vi "fault daignosis.vi"() -> ()   [LabVIEW 2023]
uses:
  <vilib>/Ngene/Deep Learning Toolkit/Toolkit/NN_Train/Controls/NN_Train_Params.ctl
  <vilib>/Ngene/Deep Learning Toolkit/Toolkit/NN_Train/Controls/NN_Train_Optimizer.ctl
  <vilib>/Ngene/Deep Learning Toolkit/Toolkit/NN_Train/Controls/NN_Train_Data_Sampling.ctl
  <vilib>/Ngene/Deep Learning Toolkit/Toolkit/NN_Train/Controls/NN_LR_Policy_Cfg.ctl
  <vilib>/Ngene/Deep Learning Toolkit/Toolkit/NN_Train/Controls/NN_LR_Policy_Type.ctl
  <vilib>/Ngene/Deep Learning Toolkit/Toolkit/NN_Train/Controls/NN_Train_Session_Data.ctl
  <vilib>/Ngene/Deep Learning Toolkit/Toolkit/NN_Network/Controls/NN_Device.ctl
  <vilib>/Ngene/Deep Learning Toolkit/Toolkit/NN_Data/API/DataSet/DataSet_Types/NN_DataSets_All(In3D_Out1D).ctl
  <vilib>/Ngene/Deep Learning Toolkit/Toolkit/NN_Data/API/DataSet/DataSet_Types/NN_DataSet(In3D_Out1D).ctl
  <vilib>/Ngene/Deep Learning Toolkit/Toolkit/NN_Data/Controls/DataRef_Types/2D/NN_Data_ref(2D_SGL).ctl
  <vilib>/Ngene/Deep Learning Toolkit/Toolkit/NN_Data/API/NN_Dims(C,H,W).ctl
  <vilib>/Ngene/Deep Learning Toolkit/Toolkit/NN_Layers/Layers/FC/Controls/NN_Layer_Config(FC).ctl
  <vilib>/Ngene/Deep Learning Toolkit/Toolkit/NN_Layers/Layers/BatchNorm/Controls/NN_BN_Params.ctl
  <vilib>/Ngene/Deep Learning Toolkit/Toolkit/NN_Activations/Controls/NN_Activation_Type.ctl
  <vilib>/Ngene/Deep Learning Toolkit/Toolkit/NN_Layers/Controls/NN_Layer_Init_Params.ctl
  <vilib>/Ngene/Deep Learning Toolkit/Toolkit/NN_Layers/Controls/NN_Layer_Weight_Init_Type.ctl
  <vilib>/Ngene/Deep Learning Toolkit/Toolkit/NN_Layers/Layers/Conv2D/Controls/NN_Layer_Config(Conv2D).ctl
  <vilib>/Ngene/Deep Learning Toolkit/Toolkit/NN_Layers/Layers/Conv2D/Controls/NN_Layer_Params(Conv2D).ctl
  <vilib>/Ngene/Deep Learning Toolkit/Toolkit/NN_Layers/Layers/Conv2D/Controls/NN_Conv2D_Padding_Type.ctl
  <vilib>/Ngene/Deep Learning Toolkit/Toolkit/NN_Layers/Layers/Pool/Controls/NN_Layer_Config(Pool).ctl
  <vilib>/Ngene/Deep Learning Toolkit/Toolkit/NN_Data/API/NN_Dims(V,H).ctl
  <vilib>/Ngene/Deep Learning Toolkit/Toolkit/NN_Layers/Layers/Activation/Controls/NN_Layer_Config(Activation).ctl
  <vilib>/Ngene/Deep Learning Toolkit/Toolkit/NN_Network/Controls/NN_Save_Before_Destroy_Options.ctl
  <vilib>/Ngene/Deep Learning Toolkit/Toolkit/NN_Layers/Layers/Input/Controls/NN_Layer_Config(Input3D).ctl
  <vilib>/Ngene/Deep Learning Toolkit/Toolkit/NN_Data/Controls/NN_Data_type.ctl
  <vilib>/Ngene/Deep Learning Toolkit/Toolkit/NN_Layers/Layers/Input/NN_Layer_Create(Input3D).vi
  <vilib>/Ngene/Deep Learning Toolkit/Toolkit/NN_Layers/Layers/Conv2D/NN_Layer_Create(Conv2D).vi
  <vilib>/Ngene/Deep Learning Toolkit/Toolkit/NN_Layers/Layers/Activation/NN_Layer_Create(Activation).vi
  <vilib>/Ngene/Deep Learning Toolkit/Toolkit/NN_Layers/Layers/Pool/NN_Layer_Create(maxPool).vi
  <vilib>/Ngene/Deep Learning Toolkit/Toolkit/NN_Layers/Layers/Flatten/NN_Layer_Create(Flatten).vi
  <vilib>/Ngene/Deep Learning Toolkit/Toolkit/NN_Layers/Layers/FC/NN_Layer_Create(FC).vi
  <vilib>/Ngene/Deep Learning Toolkit/Toolkit/NN_Layers/Layers/SoftMax/NN_Layer_Create(SoftMax).vi
  <vilib>/Ngene/Deep Learning Toolkit/Toolkit/NN_Train/Loss_Functions/NN_Set_Loss(CrossEntropy).vi
  <vilib>/Ngene/Deep Learning Toolkit/Toolkit/NN_Network/subVIs/NN_Predict/NN_Predict(In3D_Out1D).vi
  <vilib>/Ngene/Deep Learning Toolkit/Toolkit/NN_Train/Eval_Loss/NN_Eval_Test_Error_Loss/NN_Eval(In3D_Out1D).vi
  <vilib>/Ngene/Deep Learning Toolkit/Toolkit/NN_Train/Eval_Loss/NN_Calc_Cofusion_Matrix/NN_Calc_Confusion_Matrix(In3D_Out1D).vi
  <vilib>/Ngene/Deep Learning Toolkit/Toolkit/NN_Data/subVIs/Dataset_Destroy/NN_Dataset_Destroy(In3D_Out1D).vi
  <vilib>/Ngene/Deep Learning Toolkit/Toolkit/Deep_Learning_Toolkit_by_Ngene.lvlib
  <vilib>/ptbypt/NI_PtbyPt.lvlib
panel:
  out "Dataset":T1={"Train"={"Inputs Ref."=variant(refnum<data-value> refnum), "Outputs Ref."=refnum, "Dataset_Size"=0, "Dims_In"={"C"=0, "H"=0, "W"=0}, "Dims_Out"=0, "Labels"=[], "File Paths"=[], "Custom_Data"=variant}, "Validation"={"Inputs Ref."=variant(refnum<data-value> refnum), "Outputs Ref."=refnum, "Dataset_Size"=0, "Dims_In"={"C"=0, "H"=0, "W"=0}, "Dims_Out"=0, "Labels"=[], "File Paths"=[], "Custom_Data"=variant}, "Test"={"Inputs Ref."=variant(refnum<data-value> refnum), "Outputs Ref."=refnum, "Dataset_Size"=0, "Dims_In"={"C"=0, "H"=0, "W"=0}, "Dims_Out"=0, "Labels"=[], "File Paths"=[], "Custom_Data"=variant}}
  in  "Tab Control":enum32{"Model train", "Prediction"}(tab)
  in  "Start Training":bool
  in  "Train dataset path":path=path "E:/其他工作/Labviewpy联合开发/CWRU_Result/bmp_dataset_32x32/train"
  in  "NN_Train_Params":T5={"Optimizer"=enum."Adam", "Beta_1"=0.9, "Beta_2"=0.999, "Weight Decay(L1)"=0.0, "Weight Decay(L2)"=0.0001, "Data_Sampling"=enum."Random"}
  in  "Eval":bool
  out "Confusion Matrix":string[][](table)=[["1500", "0", "0", "0", "0", "0", "1.0000"], ["0", "1492", "0", "0", "8", "0", "0.9947"], ["0", "0", "1498", "0", "0", "2", "0.9987"], ["0", "0", "0", "1423", "68", "9", "0.9487"], ["0", "0", "0", "78", "1411", "11", "0.9407"], ["0", "0", "40", "3", "2", "1455", "0.9700"], ["1.0000", "1.0000", "0.9740", "0.9461", "0.9476", "0.9851", ""]]
  out "Test Loss":sgl=0.121348076 format="%#.6g"
  out "Test Error":sgl=0.024555556 format="%#.6g"
  in  "LR Update Policy":T8={"Policy_Type"=enum."Step", "LR0"=0.001, "k"=200.0, "WarmUp_Policy"=enum."Ramp", "WarmUp_Iter"=0, "WarmUp_Ratio"=1.0} {"WarmUp_Ratio" min=1; "WarmUp_Iter" min=1; "LR0" format="%.7f"}
  out "Loss Graphs":cluster{"Loss":sgl, "mean":dbl, "mean":dbl}(graph)={"Loss"=0.33578137, "mean"=0.2513088881969452, "mean"=0.3710270822048187}
  in  "Stop Training":bool
  in  "Test dataset path":path=path "E:/其他工作/Labviewpy联合开发/CWRU_Result/bmp_dataset_32x32/test"
  out "Session Data":T10={"Epochs"=251.7248, "Tot_Iter"=58998, "LR"=5e-06, "LR_iter"=58999}
  out "Time_Elapsed":dbl=138.95477960000062 format="%<%H:%M:%S>t"
  out "Training Loss":sgl=0.21247883 format="%#.6g"
  in  "NN_Device 2":T11=enum."GPU"
  in  "Datain":bool
  out "Loss":dbl=0.46153685450553894
  out "Error Rate":dbl=0.15330000221729279
  in  "NN_Device":T11=enum."GPU"
  in  "Weight File Path":path=path "E:/其他工作/Labviewpy联合开发/working/Fault_Classifier/Fault_Classifier_weights_26_05_08__18_01_11.bin"
  in  "Network Configuration File Path":path=path "E:/其他工作/Labviewpy联合开发/working/Fault_Classifier/Fault_Classifier_net_cfg_26_05_08__18_01_11.cfg"
  out "Confusion Matrix 3":string[][](table)=[["850", "4", "40", "7", "12", "1", "0", "13", "42", "31", "0.8500"], ["14", "919", "1", "1", "0", "0", "2", "2", "8", "53", "0.9190"], ["38", "1", "779", "24", "58", "29", "51", "11", "7", "2", "0.7790"], ["13", "3", "56", "658", "47", "132", "56", "20", "10", "5", "0.6580"], ["4", "3", "39", "19", "866", "10", "23", "34", "2", "0", "0.8660"], ["7", "2", "32", "101", "32", "778", "16", "26", "2", "4", "0.7780"], ["6", "3", "30", "23", "17", "12", "902", "2", "4", "1", "0.9020"], ["8", "0", "16", "24", "50", "24", "2", "870", "2", "4", "0.8700"], ["43", "13", "7", "4", "4", "3", "4", "1", "909", "12", "0.9090"], ["10", "26", "4", "8", "1", "1", "2", "4", "8", "936", "0.9360"], ["0.8560", "0.9435", "0.7759", "0.7572", "0.7967", "0.7859", "0.8526", "0.8850", "0.9145", "0.8931", ""]]
  in  "Start Prediction":bool
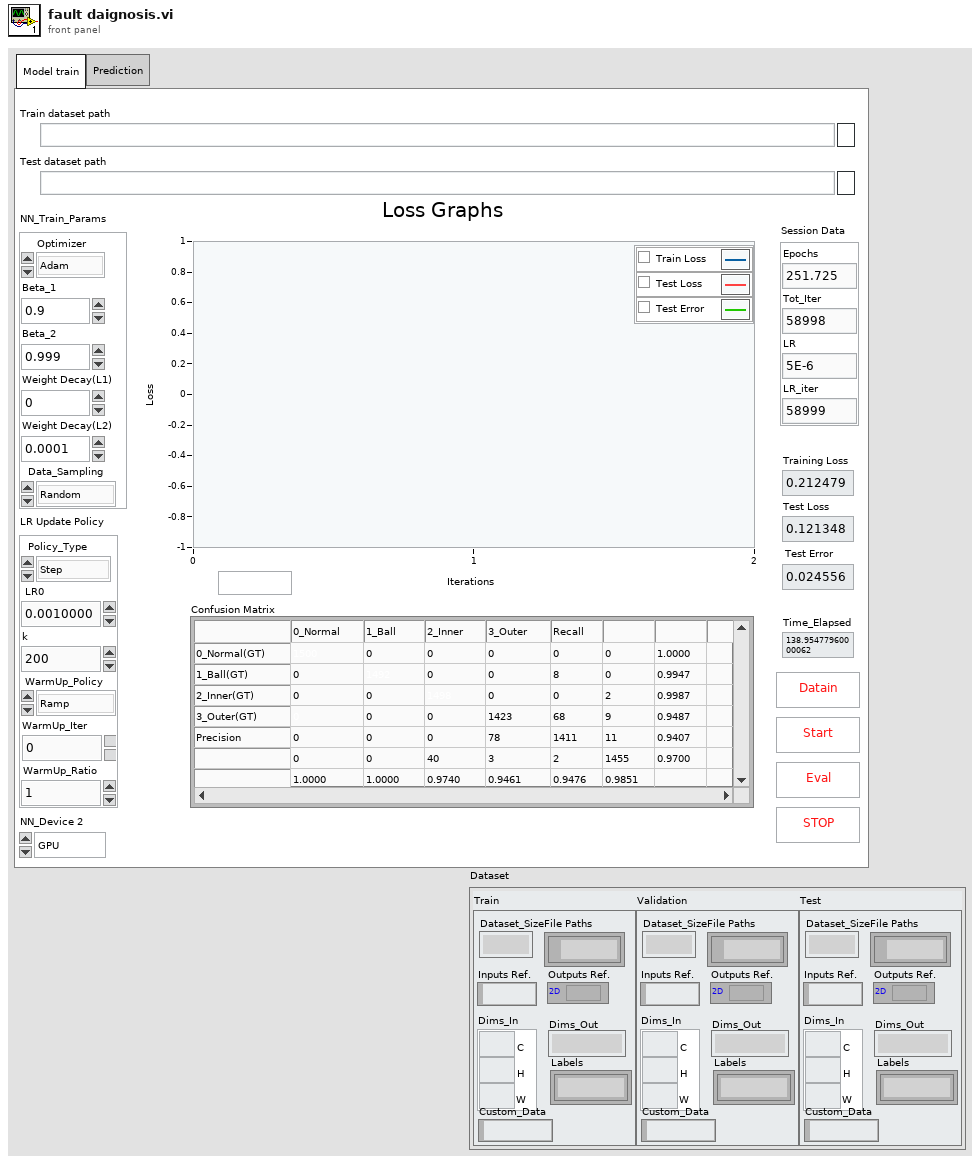
[diagram p1: front panel]
types:
  T1 = typedef "Deep_Learning_Toolkit_by_Ngene.lvlib/NN_DataSets_All(In3D_Out1D).ctl" = cluster{"Train":T2, "Validation":T2, "Test":T2}
  T2 = typedef "Deep_Learning_Toolkit_by_Ngene.lvlib/NN_DataSet(In3D_Out1D).ctl" = cluster{"Inputs Ref.":variant, "Outputs Ref.":T3, "Dataset_Size":i32, "Dims_In":T4, "Dims_Out":i32, "Labels":string[], "File Paths":path[], "Custom_Data":variant}
  T3 = typedef "Deep_Learning_Toolkit_by_Ngene.lvlib/NN_Data_ref(2D_SGL).ctl" = refnum<data-value>
  T4 = typedef "Deep_Learning_Toolkit_by_Ngene.lvlib/NN_Dims(C,H,W).ctl" = cluster{"C":i32, "H":i32, "W":i32}
  T5 = typedef "Deep_Learning_Toolkit_by_Ngene.lvlib/NN_Train_Params.ctl" = cluster{"Optimizer":T6, "Beta_1":sgl, "Beta_2":sgl, "Weight Decay(L1)":sgl, "Weight Decay(L2)":sgl, "Data_Sampling":T7}
  T6 = typedef "Deep_Learning_Toolkit_by_Ngene.lvlib/NN_Train_Optimizer.ctl" = enum16{"SGD", "Adam", "Adagrad", "Adadelta", "RMSProp", "Nesterov"}
  T7 = typedef "Deep_Learning_Toolkit_by_Ngene.lvlib/NN_Train_Data_Sampling.ctl" = enum16{"Random", "Sequential"}
  T8 = typedef "Deep_Learning_Toolkit_by_Ngene.lvlib/NN_LR_Policy_Cfg.ctl" = cluster{"Policy_Type":T9, "LR0":dbl, "k":sgl, "WarmUp_Policy":enum16{"Step", "Ramp"}, "WarmUp_Iter":i32, "WarmUp_Ratio":sgl}
  T9 = typedef "Deep_Learning_Toolkit_by_Ngene.lvlib/NN_LR_Policy_Type.ctl" = enum16{"Manual", "Step", "Exp", "1/t"}
  T10 = typedef "Deep_Learning_Toolkit_by_Ngene.lvlib/NN_Train_Session_Data.ctl" = cluster{"Epochs":sgl, "Tot_Iter":i32, "LR":sgl, "LR_iter":i32}
  T11 = typedef "Deep_Learning_Toolkit_by_Ngene.lvlib/NN_Device.ctl" = enum16{"CPU", "GPU"}
  T12 = typedef "Deep_Learning_Toolkit_by_Ngene.lvlib/NN_Layer_Config(Conv2D).ctl" = cluster{"Name":string, "Conv_Params":T13, "BN?":bool, "BN_Params":T15, "Activation":T16, "Has Bias?":bool, "Init_Params":T17, "Custom_Params":string}
  T13 = typedef "Deep_Learning_Toolkit_by_Ngene.lvlib/NN_Layer_Params(Conv2D).ctl" = cluster{"Filters":i32, "Kernel_Size":i32, "Stride":i32, "Pad_Type":T14, "Pad_Size":i32}
  T14 = typedef "Deep_Learning_Toolkit_by_Ngene.lvlib/NN_Conv2D_Padding_Type.ctl" = enum16{"Pad_Size", "Valid", "Same"}
  T15 = typedef "Deep_Learning_Toolkit_by_Ngene.lvlib/NN_BN_Params.ctl" = cluster{"epsilon":sgl, "momentum":sgl}
  T16 = typedef "Deep_Learning_Toolkit_by_Ngene.lvlib/NN_Activation_Type.ctl" = enum16{"Sigmoid", "ReLU", "LReLU", "ReLU6", "GELU", "tanh", "Swish", "Mish", "None"}
  T17 = typedef "Deep_Learning_Toolkit_by_Ngene.lvlib/NN_Layer_Init_Params.ctl" = cluster{"Init_Type":T18, "Value":sgl}
  T18 = typedef "Deep_Learning_Toolkit_by_Ngene.lvlib/NN_Layer_Weight_Init_Type.ctl" = enum16{"Const", "Uniform", "Gaussian", "Xavier"}
  T19 = typedef "Deep_Learning_Toolkit_by_Ngene.lvlib/NN_Layer_Config(Input3D).ctl" = cluster{"Name":string, "Dims":T4, "Data_Type":T20, "Shifts":sgl[], "Scales":sgl[]}
  T20 = typedef "Deep_Learning_Toolkit_by_Ngene.lvlib/NN_Data_type.ctl" = enum16{"I8", "U8", "I16", "U16", "U32 ARGB", "SGL"}
  T21 = typedef "Deep_Learning_Toolkit_by_Ngene.lvlib/NN_Save_Before_Destroy_Options.ctl" = cluster{"CFG?":bool, "Weights?":bool, "Render?":bool}
  T22 = typedef "Deep_Learning_Toolkit_by_Ngene.lvlib/NN_Layer_Config(Activation).ctl" = cluster{"Name":string, "Activation_type":T16}
  T23 = typedef "Deep_Learning_Toolkit_by_Ngene.lvlib/NN_Layer_Config(Pool).ctl" = cluster{"Name":string, "Size":T24, "Stride":T24, "Pad_Type":T14, "Pad_Size":T24}
  T24 = typedef "Deep_Learning_Toolkit_by_Ngene.lvlib/NN_Dims(V,H).ctl" = cluster{"V":i32, "H":i32}
  T25 = typedef "Deep_Learning_Toolkit_by_Ngene.lvlib/NN_Layer_Config(FC).ctl" = cluster{"Name":string, "Size":i32, "BN":bool, "BN_Params":T15, "Activation":T16, "Has Bias?":bool, "Init_Params":T17, "Custom_Params":string}
  T26 = typedef "Deep_Learning_Toolkit_by_Ngene.lvlib/NN.ctl" = cluster{"Name":string, "No of Layers":i32, "mBatch":i32, "Layers":T27[], "Dimty":T28, "Dims_In":T4, "Dims_Out":T4, "Working_Dir":path, "Train?":bool, "Train_Params":T5, "LR_Update_Policy":T8, "Session Data":T10, "Ground_truth":T29, "NNg_hdls":T30, "NN_Device":T11, "GPU Id":i32, "Labels":string[], "Loss_Type":T31, "Loss_Cfg_Prms":variant, "NNG_WS":T32, "DryRun?":bool}
  T27 = typedef "Deep_Learning_Toolkit_by_Ngene.lvlib/NN_Layer_ref.ctl" = refnum<file>
  T28 = typedef "Deep_Learning_Toolkit_by_Ngene.lvlib/NN_In_Out_Dim-ty.ctl" = enum8{"In1D_Out1D", "In3D_Out1D", "In3D_Out3D", "In3D_OutBBox"}
  T29 = typedef "Deep_Learning_Toolkit_by_Ngene.lvlib/NN_Ground_truth.ctl" = cluster{"Y":variant}
  T30 = typedef "Deep_Learning_Toolkit_by_Ngene.lvlib/nng_cuda_handles.ctl" = cluster{"cudnn":u64, "cublas":u64, "stream":u64, "curand":u64}
  T31 = typedef "Deep_Learning_Toolkit_by_Ngene.lvlib/NN_Loss_Type.ctl" = enum16{"None", "MSE", "CrossEntropy", "YOLO_v2", "YOLO_v4"}
  T32 = typedef "Deep_Learning_Toolkit_by_Ngene.lvlib/NNG_WS.ctl" = cluster{"NNG_WS_Mem":T33, "Max_WS_Size":i64}
  T33 = typedef "Deep_Learning_Toolkit_by_Ngene.lvlib/NNg_WS_Mem_DVR.ctl" = refnum<data-value>
  T34 = typedef "Deep_Learning_Toolkit_by_Ngene.lvlib/NN_Eval_Params.ctl" = cluster{"Loss":sgl, "Error":sgl}
  T35 = typedef "Deep_Learning_Toolkit_by_Ngene.lvlib/NN_Config_Params.ctl" = cluster{"Name":string, "mBatch":i32, "NN_Train_Params":T5, "LR_Decay_Policy":T8, "Labels":string[], "Loss":T36, "Max_WS_Size(B)":i64, "DryRun?":bool}
  T36 = typedef "Deep_Learning_Toolkit_by_Ngene.lvlib/NN_Loss_Config_Params.ctl" = cluster{"Loss_Type":T31, "Loss_Conf_Params":variant}
  T37 = typedef "Deep_Learning_Toolkit_by_Ngene.lvlib/NN_Layer_Config_Params.ctl" = cluster{"Layer_Type":T38, "Layer_Conf_Params":variant, "Input Layers":string[]}
  T38 = typedef "Deep_Learning_Toolkit_by_Ngene.lvlib/NN_Layer_Type.ctl" = enum16{"Input1D", "Input3D", "Conv1D", "Conv2D", "Conv2D_Adv", "MaxPool", "AvgPool", "UpSample", "DropOut3D", "ShortCut", "Concat", "SoftMax3D", "FC", "DropOut", "Softmax", "Flatten", "YOLO_v2", "YOLO_v4", "Activation", "BatchNormalization", "LayerNormalization", "Scale", "Unsupported"}
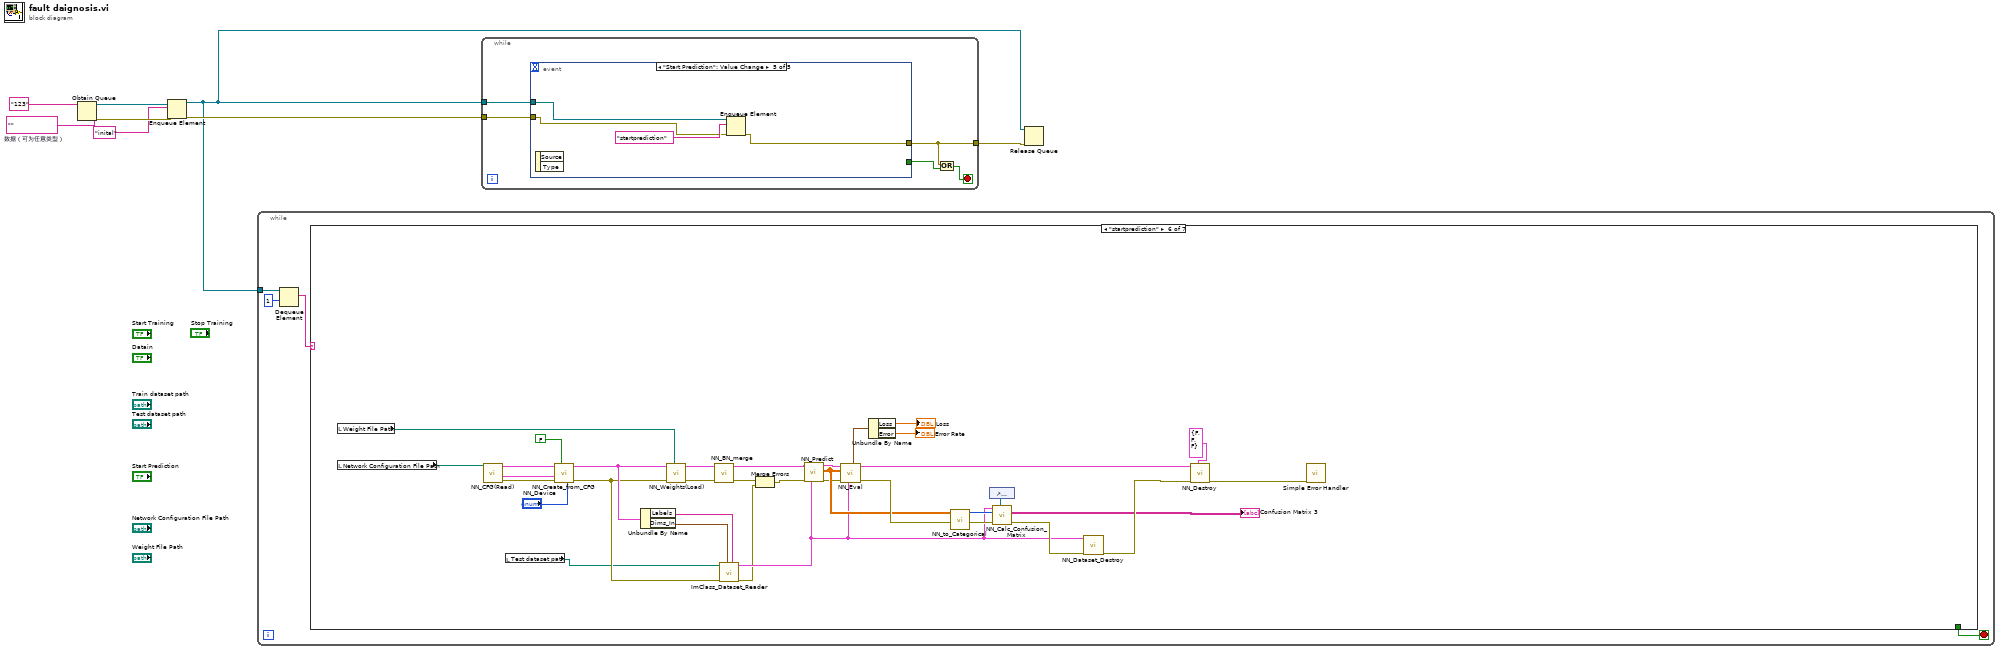
[diagram p0: block diagram]
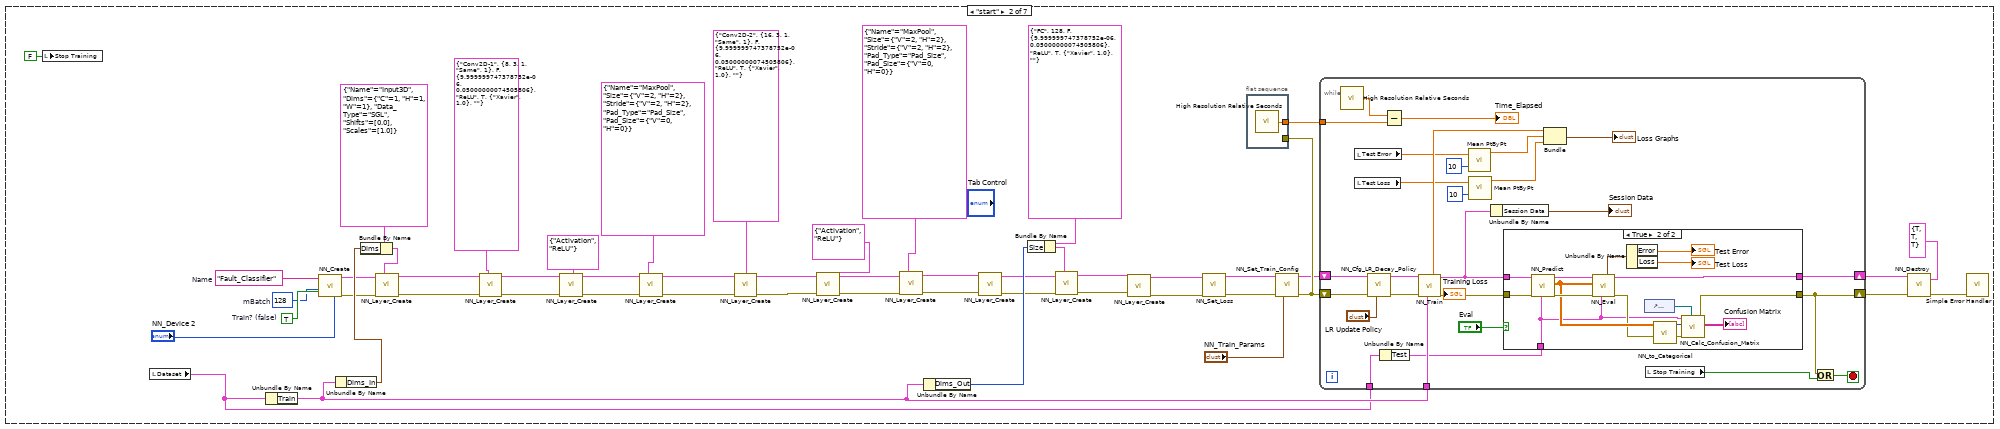
[diagram p3: hidden frame]
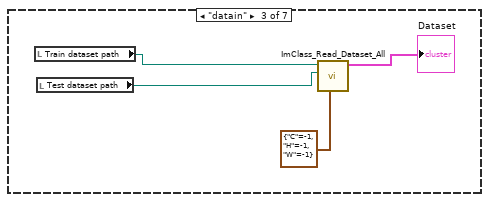
[diagram p5: hidden frame]
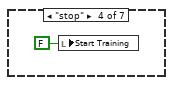
[diagram p6: hidden frame]
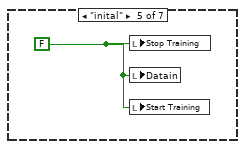
[diagram p7: hidden frame]
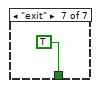
[diagram p8: hidden frame]
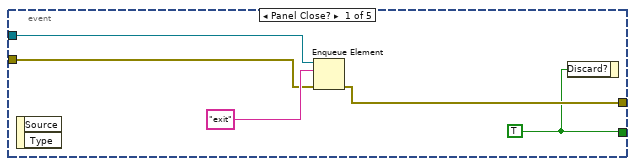
[diagram p9: hidden frame]
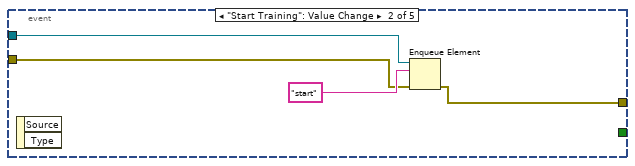
[diagram p10: hidden frame]
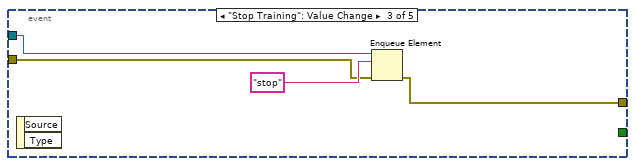
[diagram p11: hidden frame]
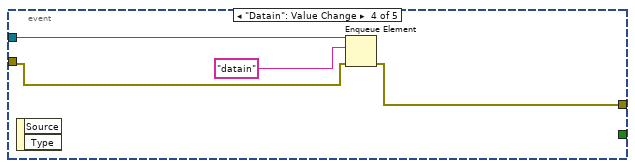
[diagram p12: hidden frame]
diagram:
  w8 = ""  # 数据（可为任意类型）
  n1 = Obtain Queue(name (unnamed)="123" ("名称（未命名）"), element data type=w8) -> (queue out=w5:refnum<queue>, error out=w6:errorcluster)  [unwired: 3 in, 1 out]
  n2 = Enqueue Element(queue=w5, element="inital", error in (no error)=w6) -> (queue out=w1:refnum<queue>, error out=w2:errorcluster)  [unwired: 1 in, 1 out]
  n3 = while {
    tunnel: w1 -> [w11]
    stop <- w9 stop-if-true
    n4 = Dequeue Element(queue=w11, timeout in ms (-1)=1 ("超时毫秒(-1)")) -> (element=w10:string)  [unwired: 1 in, 3 out]
    n5 = case shown="\"startprediction\"" w10 {
      tunnel: [_ _ _ _ _ _ TRUE] -> w9
      frame "False", Default {
      }
      frame "start" {
        w17 = TRUE  # Train? (false)
        w16 = 128  # mBatch
        w15 = "Fault_Classifier"  # Name
        n6 = local write "Stop Training"(FALSE ("Stop Training")) -> ()
        n7 = local read "Dataset"() -> (w13:T1)
        n8 = Unbundle By Name(w13) -> ("Train"=w61:T2)
        n9 = call <vilib>:"NN_Create.vi"("NN_Device"="NN_Device 2", "Train? (false)"=w17, "mBatch (1)"=w16, "Name"=w15) -> ("error out"=w29:errorcluster, "NN out"=w28:T26)  [unwired: 6 in]
        n10 = Unbundle By Name(w61) -> ("Dims_In"=w62:T4)
        n11 = Bundle By Name(cluster=T19 {"Name"="Input3D", "Dims"={"C"=1, "H"=1, "W"=1}, "Data_Type"=enum."SGL", "Shifts"=[0.0], "Scales"=[1.0]} ("Input3D_Cfg"), "Dims"=w62) -> (w63:T19)
        n12 = call-poly <vilib>:"NN_Layer_Create.vi"("Input3D_Cfg"=w63, "error in (no error)"=w29, "NN In"=w28) -> ("error out"=w50:errorcluster, "NN out"=w47:T26)  [unwired: 6 in, 1 out]
        n13 = call-poly <vilib>:"NN_Layer_Create.vi"("Conv2D_Cfg"=T12 {"Name"="Conv2D-1", "Conv_Params"={"Filters"=8, "Kernel_Size"=3, "Stride"=1, "Pad_Type"=enum."Same", "Pad_Size"=1}, "BN?"=FALSE, "BN_Params"={"epsilon"=1e-05, "momentum"=0.05}, "Activation"=enum."ReLU", "Has Bias?"=TRUE, "Init_Params"={"Init_Type"=enum."Xavier", "Value"=1.0}, "Custom_Params"=""}, "error in (no error)"=w50, "NN in"=w47) -> ("error out"=w49:errorcluster, "NN out"=w48:T26)  [unwired: 6 in, 1 out]
        n14 = call-poly <vilib>:"NN_Layer_Create.vi"("Activation_Cfg_Params"=T22 {"Name"="Activation", "Activation_type"=enum."ReLU"}, "error in (no error)"=w49, "NN in"=w48) -> ("error out"=w31:errorcluster, "NN out"=w30:T26)  [unwired: 6 in, 1 out]
        n15 = call-poly <vilib>:"NN_Layer_Create.vi"("MaxPool_Cfg"=T23 {"Name"="MaxPool", "Size"={"V"=2, "H"=2}, "Stride"={"V"=2, "H"=2}, "Pad_Type"=enum."Pad_Size", "Pad_Size"={"V"=0, "H"=0}}, "error in (no error)"=w31, "NN in"=w30) -> ("error out"=w37:errorcluster, "NN out"=w36:T26)  [unwired: 6 in, 1 out]
        n16 = call-poly <vilib>:"NN_Layer_Create.vi"("Conv2D_Cfg"=T12 {"Name"="Conv2D-2", "Conv_Params"={"Filters"=16, "Kernel_Size"=3, "Stride"=1, "Pad_Type"=enum."Same", "Pad_Size"=1}, "BN?"=FALSE, "BN_Params"={"epsilon"=1e-05, "momentum"=0.05}, "Activation"=enum."ReLU", "Has Bias?"=TRUE, "Init_Params"={"Init_Type"=enum."Xavier", "Value"=1.0}, "Custom_Params"=""}, "error in (no error)"=w37, "NN in"=w36) -> ("error out"=w34:errorcluster, "NN out"=w35:T26)  [unwired: 6 in, 1 out]
        n17 = call-poly <vilib>:"NN_Layer_Create.vi"("Activation_Cfg_Params"=T22 {"Name"="Activation", "Activation_type"=enum."ReLU"}, "error in (no error)"=w34, "NN in"=w35) -> ("error out"=w32:errorcluster, "NN out"=w33:T26)  [unwired: 6 in, 1 out]
        n18 = call-poly <vilib>:"NN_Layer_Create.vi"("MaxPool_Cfg"=T23 {"Name"="MaxPool", "Size"={"V"=2, "H"=2}, "Stride"={"V"=2, "H"=2}, "Pad_Type"=enum."Pad_Size", "Pad_Size"={"V"=0, "H"=0}}, "error in (no error)"=w32, "NN in"=w33) -> ("error out"=w39:errorcluster, "NN out"=w38:T26)  [unwired: 6 in, 1 out]
        n19 = Unbundle By Name(w61) -> ("Dims_Out"=w52:i32)
        n20 = call-poly <vilib>:"NN_Layer_Create.vi"("error in (no error)"=w39, "NN in"=w38) -> ("error out"=w41:errorcluster, "NN out"=w40:T26)  [unwired: 7 in, 1 out]
        n21 = Bundle By Name(cluster=T25 {"Name"="FC", "Size"=128, "BN"=FALSE, "BN_Params"={"epsilon"=1e-05, "momentum"=0.05}, "Activation"=enum."ReLU", "Has Bias?"=TRUE, "Init_Params"={"Init_Type"=enum."Xavier", "Value"=1.0}, "Custom_Params"=""} ("FC_Cfg"), "Size"=w52) -> (w51:T25)
        n22 = call-poly <vilib>:"NN_Layer_Create.vi"("FC_Cfg"=w51, "error in (no error)"=w41, "NN in"=w40) -> ("error out"=w43:errorcluster, "NN out"=w42:T26)  [unwired: 6 in, 1 out]
        n23 = call-poly <vilib>:"NN_Layer_Create.vi"("error in (no error)"=w43, "NN in"=w42) -> ("error out"=w45:errorcluster, "NN out"=w44:T26)  [unwired: 7 in, 1 out]
        n24 = call-poly <vilib>:"NN_Set_Loss.vi"("error in (no error)"=w45, "NN in"=w44) -> ("error out"=w54:errorcluster, "NN out"=w53:T26)  [unwired: 8 in]
        n25 = flat-sequence {
          tunnel: [w64] -> w46
          tunnel: w57 -> [_]
          frame #0 {
            n26 = call <vilib>:"High Resolution Relative Seconds.vi"() -> ("relative seconds"=w64:dbl)
          }
        }
        n27 = call <vilib>:"NN_Set_Train_Config.vi"("NN_Train_Params"="NN_Train_Params", "error in (no error)"=w54, "NN in"=w53) -> ("error out"=w57:errorcluster, "NN out"=w55:T26)  [unwired: 7 in]
        n28 = while {
          tunnel: w46 -> [w90]
          shift-right: [w82] -> w58
          shift-left: w55 -> [w89]
          shift-right: [w71] -> w59
          shift-left: w57 -> [w88]
          tunnel: w61 -> [w85]
          tunnel: w13 -> [w84]
          stop <- w70 stop-if-true
          n29 = call <vilib>:"High Resolution Relative Seconds.vi"() -> ("relative seconds"=w91:dbl)
          n30 = local read "Test Error"() -> (w77:sgl)
          n31 = local read "Test Loss"() -> (w76:sgl)
          n32 = call <vilib>:"NN_Cfg_LR_Decay_Policy.vi"("LR_Decay_Params"="LR Update Policy", "error in (no error)"=w88, "NN in"=w89) -> ("error out"=w86:errorcluster, "NN out"=w87:T26)  [unwired: 7 in]
          n33 = Unbundle By Name(w84) -> ("Test"=w69:T2)
          n34 = Subtract(x=w91, y=w90) -> (x-y=→"Time_Elapsed":dbl)
          n35 = call <vilib>:"NN_Train.vi"("Train Dataset"=w85, "error in (no error)"=w86, "NN in"=w87) -> ("error out"=w83:errorcluster, "NN out"=w68:T26, "Loss"=w79:sgl)  [unwired: 3 in, 3 out]
          n36 = call <vilib>:"Mean PtByPt.vi"("x"=w77, "sample length"=10) -> ("mean"=w75:dbl)  [unwired: 2 in, 1 out]
          n37 = call <vilib>:"Mean PtByPt.vi"("x"=w76, "sample length"=10) -> ("mean"=w74:dbl)  [unwired: 2 in, 1 out]
          n38 = Unbundle By Name(w68) -> ("Session Data"=→"Session Data":T10)
          n39 = case shown="True" "Eval" {
            tunnel: w68 -> [w93 w107]
            tunnel: w83 -> [w92 w106]
            tunnel: [w93 w105] -> w82
            tunnel: [w92 w100] -> w71
            tunnel: w69 -> [_ w94]
            frame False {
            }
            frame True {
              n40 = call-poly <vilib>:"NN_Predict.vi"("Dataset"=w94, "error in (no error)"=w106, "NN in"=w107) -> ("error out"=w108:errorcluster, "Predictions"=w103:sgl[][], "NN out"=w104:T26)  [unwired: 6 in]
              n41 = call-poly <vilib>:"NN_Eval.vi"("Dataset"=w94, "error in (no error)"=w108, "Predictions"=w103, "NN in"=w104) -> ("error out"=w101:errorcluster, "NN out"=w105:T26, "NN_Eval_Params"=w97:T34)  [unwired: 4 in, 1 out]
              n42 = Unbundle By Name(w97) -> ("Error"=→"Test Error":sgl, "Loss"=→"Test Loss":sgl)
              n43 = control-ref of="Confusion Matrix"() -> (w98:refnum<vi>)
              n44 = call <vilib>:"NN_to_Categorical.vi"("Prediction"=w103) -> ("Label_Idx"=w102:i32[])  [unwired: 10 in]
              n45 = call-poly <vilib>:"NN_Calc_Confusion_Matrix.vi"("Confusion Matrix (Table) ref."=w98, "error in (no error)"=w101, "Predictions"=w102, "Dataset"=w94) -> ("error out"=w100:errorcluster, "Confusion Matrix (Table)"=→"Confusion Matrix":string[][])  [unwired: 3 in, 3 out]
            }
          }
          n46 = Bundle("Loss"=w79, "mean"=w75, "mean"=w74) -> (→"Loss Graphs":cluster{"Loss":sgl, "mean":dbl, "mean":dbl})  [unwired: 1 in]
          n47 = local read "Stop Training"() -> (w65:bool)
          n48 = Or(x=w71, y=w65) -> (x .or. y?=w70:bool)
        }
        n49 = call <vilib>:"NN_Destroy.vi"("Save (T, T, T)"=T21 {"CFG?"=TRUE, "Weights?"=TRUE, "Render?"=TRUE}, "error in (no error)"=w59, "NN in"=w58) -> ("error out"=w60:errorcluster)  [unwired: 7 in, 1 out]
        n50 = call <vilib>:"Simple Error Handler.vi"("error in (no error)"=w60) -> ()  [unwired: 4 in, 5 out]
      }
      frame "datain" {
        n51 = local read "Train dataset path"() -> (w111:path)
        n52 = local read "Test dataset path"() -> (w110:path)
        n53 = call "ImClass_Read_Dataset_All.vi"("Dims(C,H,W)"=T4 {"C"=-1, "H"=-1, "W"=-1}, "Test Path"=w110, "Train Path"=w111) -> ("Dataset"=→"Dataset":T1)  [unwired: 7 in, 1 out]
      }
      frame "stop" {
        n54 = local write "Start Training"(FALSE ("Start Training")) -> ()
      }
      frame "inital" {
        w114 = FALSE ("Stop Training")
        n55 = local write "Stop Training"(w114) -> ()
        n56 = local write "Datain"(w114) -> ()
        n57 = local write "Start Training"(w114) -> ()
      }
      frame "startprediction" {
        n58 = local read "Weight File Path"() -> (w115:path)
        n59 = local read "Network Configuration File Path"() -> (w116:path)
        n60 = call <vilib>:"NN_CFG(Read).vi"("CFG file path"=w116) -> ("error out"=w123:errorcluster, "Net_Cfg"=w122:T35, "Layer_Cfg"=w124:T37[])  [unwired: 8 in]
        n61 = local read "Test dataset path"() -> (w117:path)
        n62 = call <vilib>:"NN_Create_from_CFG.vi"("NN_Device"="NN_Device", "Train? (false)"=FALSE, "error in (no error)"=w123, "Net_Cfg"=w122, "Layer_Cfg"=w124) -> ("error out"=w129:errorcluster, "NN out"=w134:T26)  [unwired: 5 in]
        n63 = Unbundle By Name(w134) -> ("Labels"=w135:string[], "Dims_In"=w136:T4)
        n64 = call <vilib>:"NN_Weights(Load).vi"("Weight File Path"=w115, "error in (no error)"=w129, "NN in"=w134) -> ("error out"=w126:errorcluster, "NN out"=w125:T26)  [unwired: 7 in]
        n65 = call <vilib>:"NN_BN_merge.vi"("error in (no error)"=w126, "NN in"=w125) -> ("error out"=w128:errorcluster, "NN out"=w127:T26)  [unwired: 8 in]
        n66 = call "ImClass_Dataset_Reader.vi"("Unique labels"=w135, "Dims(C,H,W)"=w136, "error in (no error)"=w129, "Image Foldr Path"=w117) -> ("error out"=w131:errorcluster, "NN_DataSet(In3D_OutBBox)"=w133:T2)  [unwired: 6 in]
        n67 = Merge Errors(w128, w131) -> (w130:errorcluster)
        n68 = call-poly <vilib>:"NN_Predict.vi"("Dataset"=w133, "error in (no error)"=w130, "NN in"=w127) -> ("error out"=w141:errorcluster, "Predictions"=w143:sgl[][], "NN out"=w140:T26)  [unwired: 6 in]
        n69 = call-poly <vilib>:"NN_Eval.vi"("Dataset"=w133, "error in (no error)"=w141, "Predictions"=w143, "NN in"=w140) -> ("error out"=w148:errorcluster, "NN out"=w121:T26, "NN_Eval_Params"=w145:T34)  [unwired: 4 in, 1 out]
        n70 = Unbundle By Name(w145) -> ("Loss"=→"Loss":sgl, "Error"=→"Error Rate":sgl)
        n71 = call <vilib>:"NN_to_Categorical.vi"("Prediction"=w143) -> ("Label_Idx"=w142:i32[])  [unwired: 10 in]
        n72 = control-ref of="Confusion Matrix 3"() -> (w139:refnum<vi>)
        n73 = call-poly <vilib>:"NN_Calc_Confusion_Matrix.vi"("Confusion Matrix (Table) ref."=w139, "error in (no error)"=w148, "Predictions"=w142, "Dataset"=w133) -> ("error out"=w144:errorcluster, "Confusion Matrix (Table)"=→"Confusion Matrix 3":string[][])  [unwired: 3 in, 3 out]
        n74 = call-poly <vilib>:"NN_Dataset_Destroy.vi"("error in (no error)"=w144, "Dataset(In3D_Out1D)"=w133) -> ("error out"=w132:errorcluster)  [unwired: 9 in]
        n75 = call <vilib>:"NN_Destroy.vi"("Save (T, T, T)"=T21 {"CFG?"=FALSE, "Weights?"=FALSE, "Render?"=FALSE} ("Save_Config"), "error in (no error)"=w132, "NN in"=w121) -> ("error out"=w138:errorcluster)  [unwired: 7 in, 1 out]
        n76 = call <vilib>:"Simple Error Handler.vi"("error in (no error)"=w138) -> ()  [unwired: 4 in, 5 out]
      }
      frame "exit" {
      }
    }
  }
  n77 = while {
    tunnel: w2 -> [w153]
    tunnel: [w152] -> w3
    tunnel: w1 -> [w150]
    stop <- w154 stop-if-true
    n78 = event shown="[4] \"Start Prediction\": Value Change" {
      selector: _ -> [_ _ _ _ _]
      dyn-events: _ -> [_ _ _ _ _]
      timeout: _ -> [_ _ _ _ _]
      tunnel: w153 -> [w158 w161 w165 w169 w173]
      tunnel: [w157 w160 w164 w168 w172] -> w152
      tunnel: [w155 _ _ _ _] -> w151
      tunnel: w150 -> [w156 w162 w167 w170 w174]
      event Panel Close? {
        w155 = TRUE
        n79 = event-data() -> ()  [unwired: 1 in, 2 out]
        n80 = Enqueue Element(queue=w156, element="exit", error in (no error)=w158) -> (error out=w157:errorcluster)  [unwired: 1 in, 2 out]
        n81 = event-data("Discard?"=w155) -> ()  [unwired: 1 in, 1 out]
      }
      event "Start Training": Value Change {
        n82 = event-data() -> ()  [unwired: 1 in, 2 out]
        n83 = Enqueue Element(queue=w162, element="start", error in (no error)=w161) -> (error out=w160:errorcluster)  [unwired: 1 in, 2 out]
      }
      event "Stop Training": Value Change {
        n84 = event-data() -> ()  [unwired: 1 in, 2 out]
        n85 = Enqueue Element(queue=w167, element="stop", error in (no error)=w165) -> (error out=w164:errorcluster)  [unwired: 1 in, 2 out]
      }
      event "Datain": Value Change {
        n86 = event-data() -> ()  [unwired: 1 in, 2 out]
        n87 = Enqueue Element(queue=w170, element="datain", error in (no error)=w169) -> (error out=w168:errorcluster)  [unwired: 1 in, 2 out]
      }
      event "Start Prediction": Value Change {
        n88 = event-data() -> ()  [unwired: 1 in, 2 out]
        n89 = Enqueue Element(queue=w174, element="startprediction", error in (no error)=w173) -> (error out=w172:errorcluster)  [unwired: 1 in, 2 out]
      }
    }
    n90 = Or(x=w152, y=w151) -> (x .or. y?=w154:bool)
  }
  n91 = Release Queue(queue=w1, error in (no error)=w3) -> ()  [unwired: 1 in, 3 out]
